vi "sub_Resamp_Demod_Shell.vi"(4 "Rx IQ Sampling\nRate [s/sec]":dbl, 5 "PSK Init Parameters":T2, 8 "Input Packets":cluster{"Packets":cdb[][], "Enable?":bool}) -> (0 "Synch Found?":bool, 1 "recovered complex waveform":T1[](array[typedef]) {"Y" format="%.3f"; "dt" format="%^.2e"; "t0" format="%.4f"}, 3 "Output Bitstream":cluster{"bit stream":i8[][], "Enable?":bool})   [LabVIEW 2015]
uses:
  <vilib>/addons/Modulation/Analog/controls/Complex Data Waveform.ctl
  <vilib>/addons/Modulation/niAMT.lvlib
panel:
  in  "error in (no error)":errorcluster
  out "error out":errorcluster
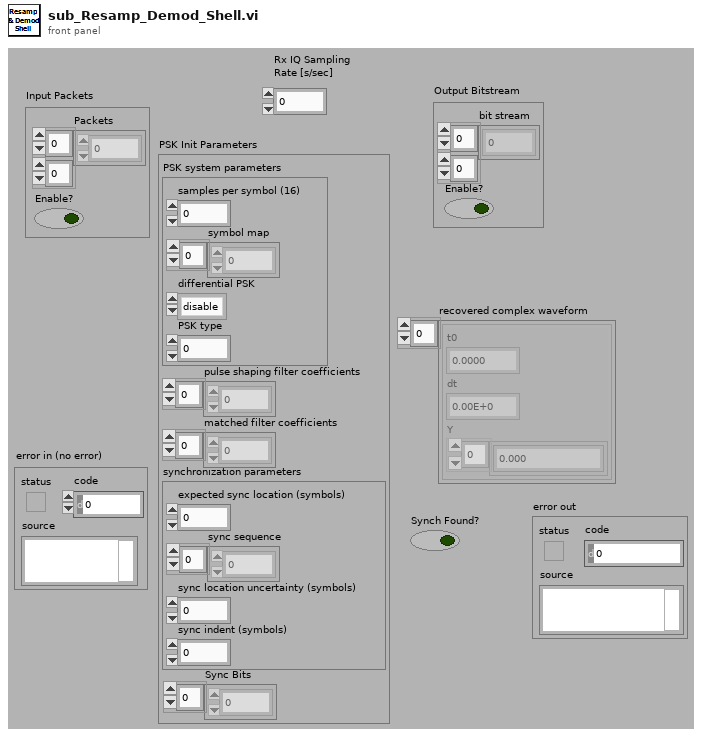
[diagram p1: front panel]
types:
  T1 = typedef "niAMT.lvlib/Complex Data Waveform.ctl" = cluster{"t0":dbl, "dt":dbl, "Y":cdb[]}
  T2 = cluster{"PSK system parameters":cluster{"samples per symbol (16)":i32, "symbol map":cdb[], "differential PSK":enum16{"disable", "enable"}, "PSK type":u16}, "pulse shaping filter coefficients":dbl[], "matched filter coefficients":dbl[], "synchronization parameters":cluster{"expected sync location (symbols)":i32, "sync sequence":cdb[], "sync location uncertainty (symbols)":i32, "sync indent (symbols)":i32}, "Sync Bits":i8[]}
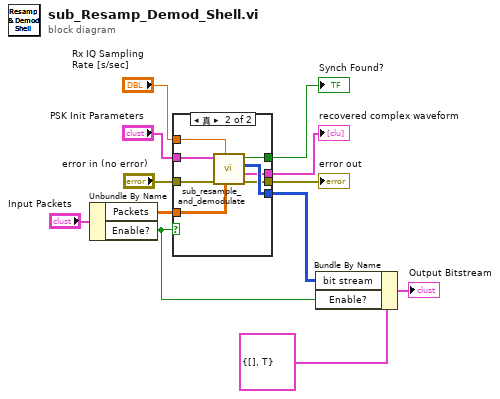
[diagram p0: block diagram]
diagram:
  n1 = Unbundle By Name("Input Packets") -> ("Packets"=w4:cdb[][], "Enable?"=w3:bool)
  n2 = case shown="真" w3 {
    tunnel: "Rx IQ Sampling\nRate [s/sec]" -> [_ w16]
    tunnel: [_ w20] -> w7
    tunnel: "PSK Init Parameters" -> [_ w19]
    tunnel: [_ w18] -> w6
    tunnel: [_ w17] -> w10
    tunnel: [_ w15] -> w9
    tunnel: "error in (no error)" -> [_ w14]
    tunnel: w4 -> [_ w13]
    frame False {
    }
    frame True {
      n3 = call "sub_resample_and_demodulate.vi"("packet_arr"=w13, "Rx IQ Sampling\nRate [s/sec]"=w16, "error in (no error)"=w14, "PSK Init Parameters"=w19) -> ("error out"=w15:errorcluster, "recovered complex waveform"=w17:T1[], "output bit stream"=w20:i8[][], "Sync Found"=w18:bool)  [unwired: 2 in]
    }
  }
  "Synch Found?" <- w6
  "recovered complex waveform" <- w10
  "error out" <- w9
  n4 = Bundle By Name(cluster=cluster{"bit stream":i8[][], "Enable?":bool} {"bit stream"=[], "Enable?"=TRUE} ("Output Bitstream"), "bit stream"=w7, "Enable?"=w3) -> (→"Output Bitstream":cluster{"bit stream":i8[][], "Enable?":bool})
